vi "Configure Display.vi"(8 "Error In (no error)":errorcluster, 9 "Channel 2 Display (0: Y)":u16(ring) items=["Y", "Phi", "Y noise [Volts]", "Y noise [dBm]", "AUX IN 2"], 10 "Channel 1 Display (0: X)":u16(ring) items=["X", "R [Volts rms]", "R [dBm]", "X noise", "AUX IN 1"], 11 "VISA Resource Name":refnum<visa-resource-name>) -> (0 "Error Out":errorcluster, 3 "VISA Resource Name Out":refnum<visa-resource-name>)   [LabVIEW 2010, in "Stanford Research 844.lvlib"]
doc: "This VI configures display."
uses:
  <instrlib>/Stanford Research 844/Stanford Research 844.lvlib
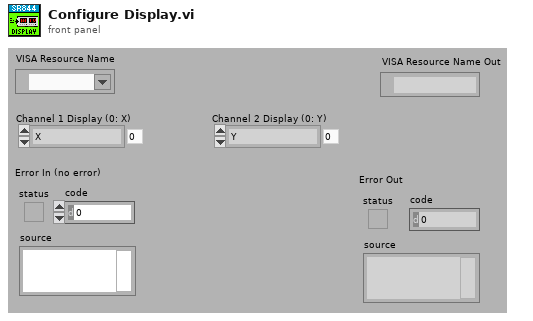
[diagram p1: front panel]
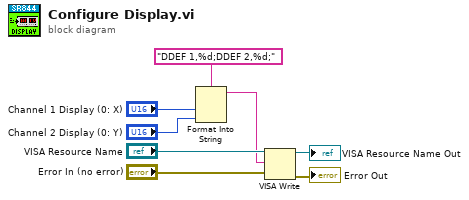
[diagram p0: block diagram]
diagram:
  n1 = Format Into String(format string="DDEF 1,%d;DDEF 2,%d;", "Channel 1 Display (0: X)", "Channel 2 Display (0: Y)") -> (resulting string=w1:string)  [unwired: 2 in, 1 out]
  n2 = VISA Write(VISA resource name="VISA Resource Name", write buffer=w1, error in (no error)="Error In (no error)") -> (VISA resource name out=→"VISA Resource Name Out":refnum<visa-resource-name>, error out=→"Error Out":errorcluster)  [unwired: 1 out]
